vi "Dequeue and Save ActrosRef.vi"(8 "error in (no error)":errorcluster, 11 "ModuleAbstract in":refnum<class "ModuleAbstract.lvclass">) -> (0 "error out":errorcluster, 3 "ModuleAbstract out":refnum<class "ModuleAbstract.lvclass">)   [LabVIEW 2019, in "ModuleAbstract.lvlib" / "ModuleAbstract.lvclass"]
uses:
  ModuleAbstract.lvclass
  TypeDef/SelfQueue Msg.ctl
  Containers/ActorRefContainer/ActorRefContainer.lvclass
  ModuleAbstract.lvclass/ModuleAbstract.ctl
  624c2b7c-be1a-4985-88e8-4c408afb5df5.vi
  <vilib>/Utility/Data Type/Get Numeric Information.vi
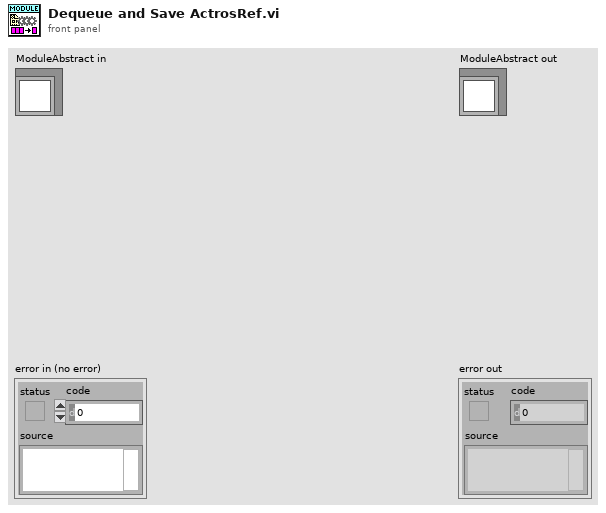
[diagram p1: front panel]
types:
  T1 = typedef "ModuleAbstract.lvlib/ModuleAbstract.lvclass/SelfQueue Msg.ctl" = enum16{"Read All Actors REF"}
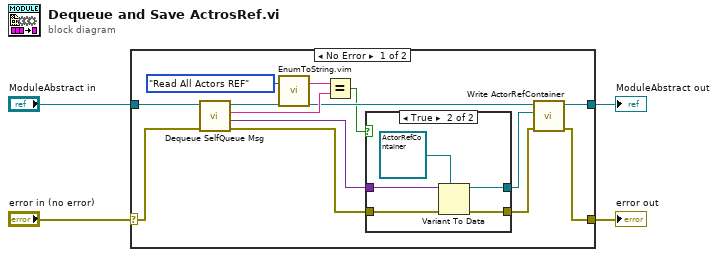
[diagram p0: block diagram]
diagram:
  n1 = case shown="No Error" "error in (no error)" {
    selector: "error in (no error)" -> [w16 w25]
    tunnel: [w5 w25] -> w3
    tunnel: [w8 w24] -> w1
    tunnel: "ModuleAbstract in" -> [w17 w24]
    frame No Error {
      n2 = call "Dequeue SelfQueue Msg.vi"("error in (no error)"=w16, "ModuleAbstract in"=w17) -> ("error out"=w9:errorcluster, "Message Data"=w10:variant, "Message"=w13:string, "ModuleAbstract out"=w12:refnum<class "ModuleAbstract.lvclass">)  [unwired: 6 in]
      n3 = call "EnumToString.vim"("Enum"=SelfQueue_Msg."Read All Actors REF" ("SelfQueue Msg")) -> ("Enum Value"=w14:string)  [unwired: 16 in, 2 out]
      n4 = Equal?(x=w14, y=w13) -> (x = y?=w11:bool)
      n5 = case shown="True" w11 {
        tunnel: w10 -> [_ w23]
        tunnel: w9 -> [w18 w22]
        tunnel: [_ w20] -> w7
        tunnel: [w18 w19] -> w6
        frame False {
        }
        frame True {
          n6 = Variant To Data(error in=w22, type=refnum<class "ActorRefContainer.lvclass"> refnum ("ActorRefContainer.lvlib:ActorRefContainer.lvclass"), Variant=w23) -> (data=w20:refnum<class "ActorRefContainer.lvclass">, error out=w19:errorcluster)
        }
      }
      n7 = call "Write ActorRefContainer.vi"("error in (no error)"=w6, "ActorRefContainer"=w7, "ModuleAbstract in"=w12) -> ("error out"=w5:errorcluster, "ModuleAbstract out"=w8:refnum<class "ModuleAbstract.lvclass">)  [unwired: 7 in]
    }
    frame Error {
    }
  }
  "error out" <- w3
  "ModuleAbstract out" <- w1
